vi "Get Pixel Intensity Array Left To Calibrate Cams_Luan2024.05.01.vi"(4 "error in (no error)":errorcluster, 5 "Selected line":i32=300, 6 "X Step Size":i32=-200, 7 "Image":T1(plugin-control)) -> (0 "error out":errorcluster, 1 "Intensity vs Pixel":u8[](graph), 2 "Image 2":T1(plugin-control), 3 "ROI Descriptor":T2 {"Contours"."Type" items=["No Selection", "Point", "Line", "Rectangle", "Oval", "Polygon", "Freehand Region", "Annulus", "Unused2", "Unused3", "Broken Line", "Freehand Line", "Rotated Rectangle"]})   [LabVIEW 2023]
uses:
  <vilib>/vision/NI_Vision_Development_Module.lvlib
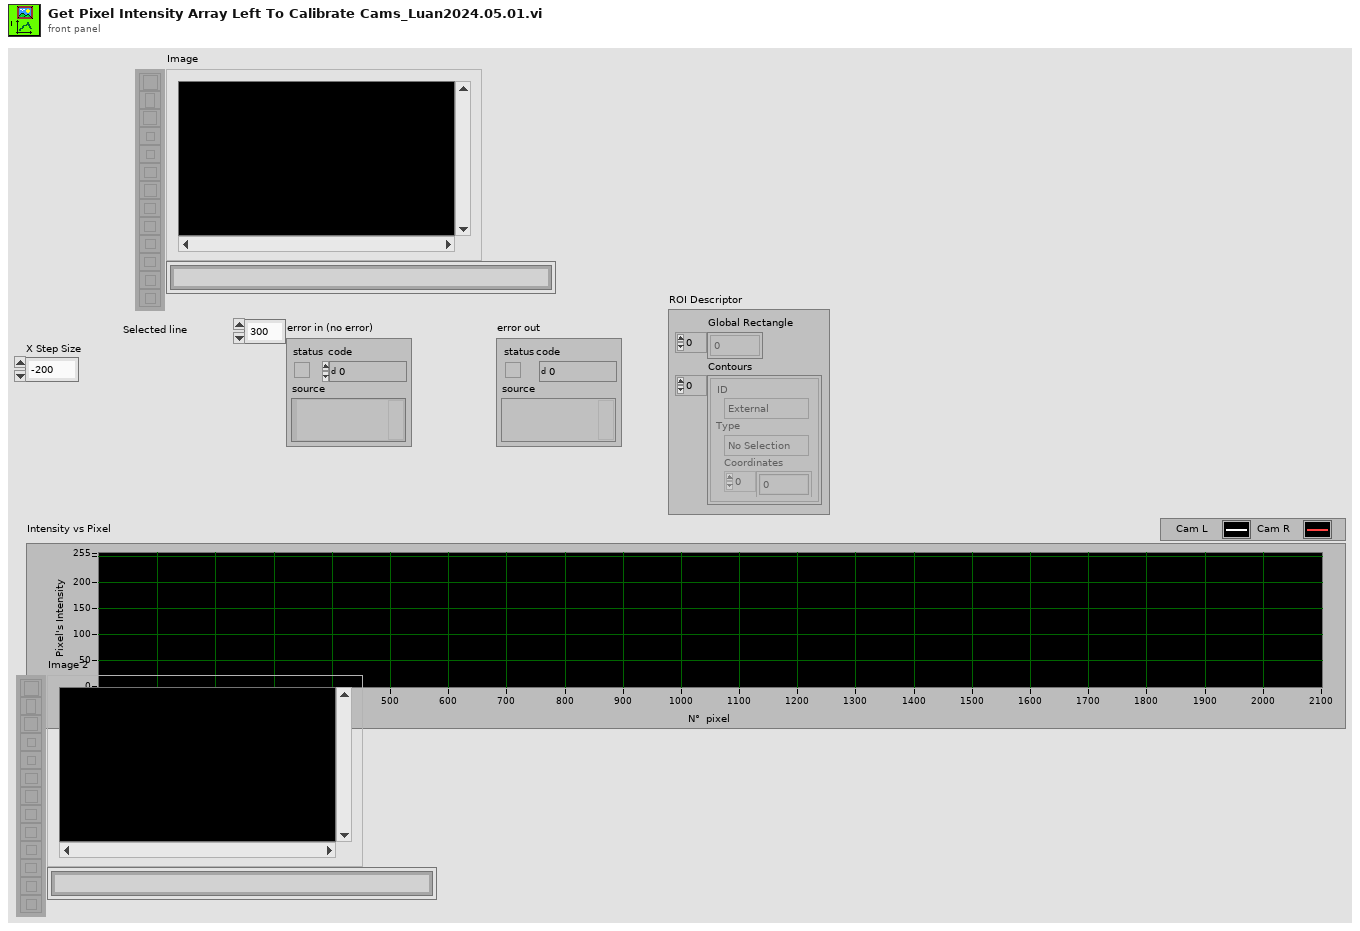
[diagram p1: front panel]
types:
  T1 = typedef "IMAQ Image.ctl" = refnum<image>
  T2 = typedef "ROI Descriptor" = cluster{"Global Rectangle":i32[], "Contours":cluster{"ID":enum32{"External", "Internal"}, "Type":u32, "Coordinates":i32[]}[]}
  T3 = typedef "IMAQ Line" = cluster{"Start X":i32, "Start Y":i32, "End X":i32, "End Y":i32}
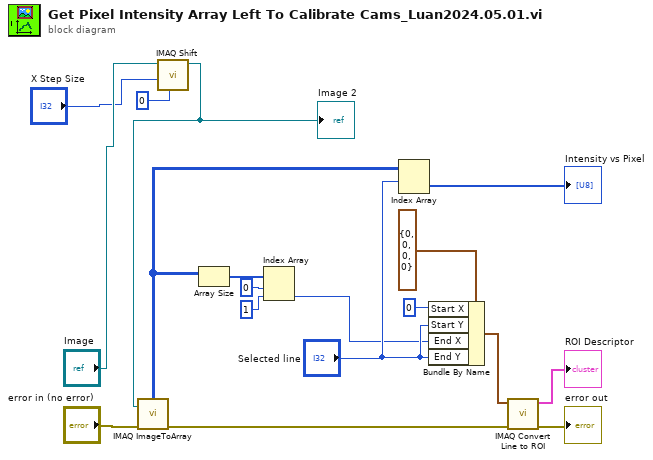
[diagram p0: block diagram]
diagram:
  n1 = call "IMAQ Shift"("YOffset"=0, "XOffset"="X Step Size", "Image Src"="Image") -> ("Image Dst Out"=w2:T1)  [unwired: 7 in, 1 out]
  "Image 2" <- w2
  n2 = call "IMAQ ImageToArray"("error in (no error)"="error in (no error)", "Image"=w2) -> ("error out"=w13:errorcluster, "Image Pixels (U8)"=w6:u8[][])  [unwired: 2 in, 3 out]
  n3 = Array Size(array=w6) -> (size(s)=w7:i32[])
  n4 = Index Array(array=w7, index #1=0 ("index"), index #2=1 ("index")) -> (element #2=w5:i32)  [unwired: 1 out]
  n5 = Index Array(array=w6, index (row)="Selected line") -> (element=→"Intensity vs Pixel":u8[])  [unwired: 1 in]
  n6 = Bundle By Name(cluster=T3 {"Start X"=0, "Start Y"=0, "End X"=0, "End Y"=0} ("Line"), "Start X"=0, "Start Y"="Selected line", "End X"=w5, "End Y"="Selected line") -> (w11:T3)
  n7 = call "IMAQ Convert Line to ROI"("error in (no error)"=w13, "Line"=w11) -> ("error out"=→"error out":errorcluster, "ROI Descriptor"=→"ROI Descriptor":T2)  [unwired: 7 in]
